vi "Lockin SR830.vi"(8 "error in (no error)":errorcluster, 10 "Is SR830? (T)":bool=TRUE, 11 "Lockin SR830 in":refnum<class "Lockin SR830.lvclass">) -> (0 "error out":errorcluster, 3 "Lockin SR830 out":refnum<class "Lockin SR830.lvclass">)   [LabVIEW 2012, in "Lockin SR830.lvclass"]
uses:
  Lockin SR830.lvclass
  Lockin SR830.lvclass/Lockin SR830.ctl
  Global/GPIB Numbers.vi
  Utility Classes/Readable/Readable.lvclass
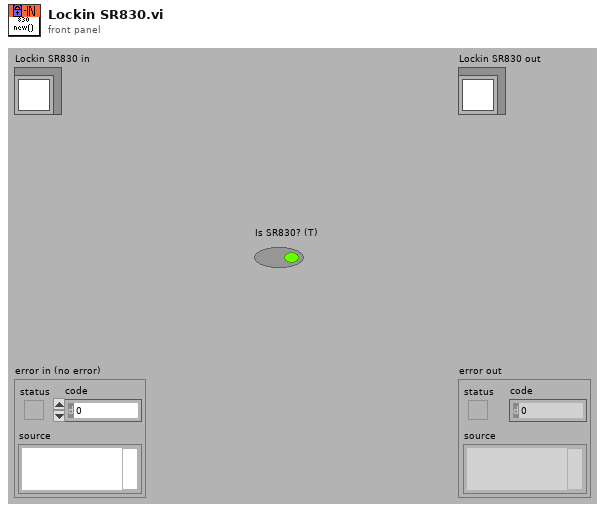
[diagram p1: front panel]
types:
  T1 = typedef "GPIB Type Def.ctl" = cluster{"Name":string, "bus":dbl, "GPIB":dbl, "GPIB as string":string, "byte":i32, "VISA Resource Name":refnum<visa-resource-name>}
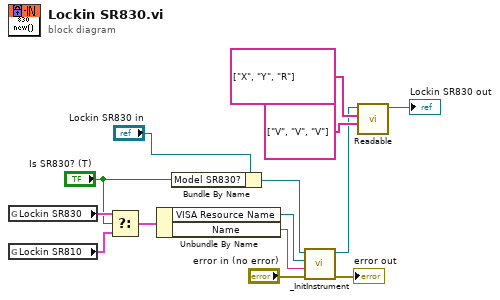
[diagram p0: block diagram]
diagram:
  n1 = global read "GPIB Numbers.vi" "Lockin SR830"() -> (w8:T1)
  n2 = global read "GPIB Numbers.vi" "Lockin SR810"() -> (w9:T1)
  n3 = Select(t=w8, s="Is SR830? (T)", f=w9) -> (s? t:f=w7:T1)
  n4 = Unbundle By Name(w7) -> ("VISA Resource Name"=w5:refnum<visa-resource-name>, "Name"=w10:string)
  n5 = Bundle By Name(cluster="Lockin SR830 in", "Model SR830?"="Is SR830? (T)") -> (w13:refnum<class "Lockin SR830.lvclass">)
  n6 = call-dynamic "_InitInstrument.vi"("error in (no error)"="error in (no error)", "Name"=w10, "VISA Resource Name"=w5, "Instrument in"=w13) -> ("error out"=→"error out":errorcluster, "Instrument out"=w2:refnum<class "Lockin SR830.lvclass">)  [unwired: 2 in, 4 out]
  n7 = call "Readable.vi"("Channel Units"=string[] ["V", "V", "V"], "Channel Names"=string[] ["X", "Y", "R"], "Readable in"=w2) -> ("Readable out"=→"Lockin SR830 out":refnum<class "Lockin SR830.lvclass">)  [unwired: 7 in, 1 out]
